vi "Button.vi"(10 "Button":bool, 11 "Dev Panel in":refnum<class "Dev Panel.lvclass">) -> (0 "error out":errorcluster)   [LabVIEW 2021, in "Dev Panel.lvclass"]
uses:
  Dev Panel.lvclass
  Dev Panel.lvclass/Dev Panel.ctl
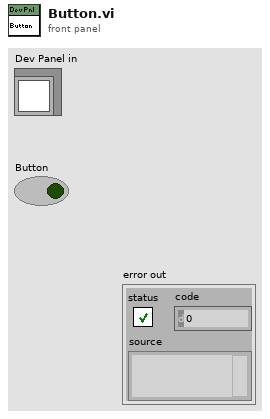
[diagram p1: front panel]
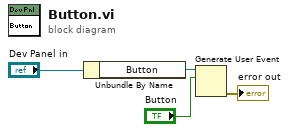
[diagram p0: block diagram]
diagram:
  n1 = Unbundle By Name("Dev Panel in") -> ("Button"=w3:refnum<user-event>)
  n2 = Generate User Event(user event=w3, event data cluster="Button") -> (error out=→"error out":errorcluster)  [unwired: 2 in, 1 out]
